vi "GetFeaturesToRegister.vi"(6 "Supported Metrics":string[](array[string]), 7 "high rate":bool, 8 "error in (no error)":errorcluster, 10 "group":string, 11 "channels":T1[](array[typedef])) -> (0 "error out":errorcluster, 2 "atleast one":bool, 3 "register trend":T5)   [LabVIEW 2017, in "McsaAnalysisHighRate.lvlib"]
uses:
  <vilib>/addons/InsightCM/Devices/Shared/Mcsa/McsaAnalysisHighRate/McsaAnalysisHighRate.lvlib
  <vilib>/addons/InsightCM/Devices/Shared/Common/DataEventCreator/controls/RegisterTrendPoints.ctl
  <vilib>/addons/InsightCM/Devices/Shared/Common/DataEventCreator/controls/Registry_Trend.ctl
  <vilib>/addons/InsightCM/Utilities/Analysis/MCSA/controls/McsaChannel.ctl
  <vilib>/addons/InsightCM/Utilities/Analysis/Shared/controls/Feature.ctl
  <vilib>/addons/InsightCM/Utilities/Analysis/Shared/controls/AmplitudeScale.ctl
  <vilib>/addons/InsightCM/MessageBus/Base/controls/KeyValuePair.ctl
  <vilib>/addons/InsightCM/Devices/Shared/Common/DataEventCreator/DataEventCreator.lvlib
  <vilib>/addons/InsightCM/Utilities/Analysis/Shared/AnalysisHelper.lvlib
  <vilib>/addons/InsightCM/Utilities/Analysis/MCSA/McsaAnalysisFunctions.lvlib
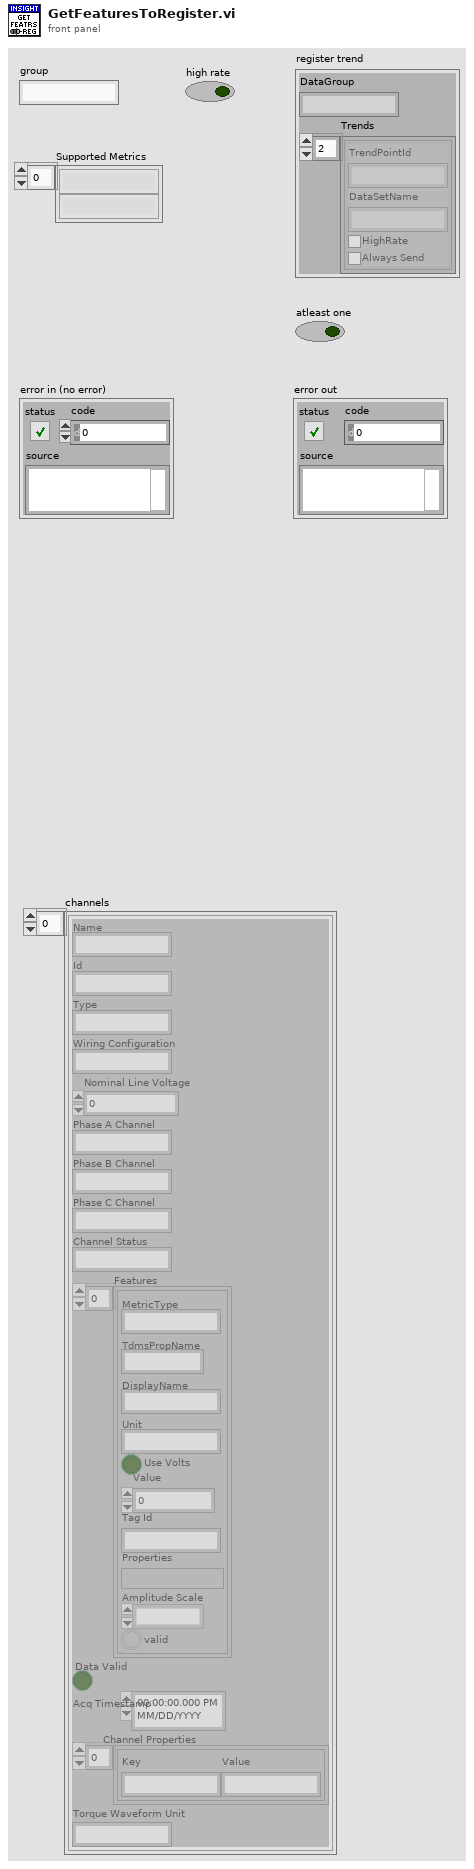
[diagram p1: front panel]
types:
  T1 = typedef "McsaAnalysisFunctions.lvlib/McsaChannel.ctl" = cluster{"Name":string, "Id":string, "Type":string, "Wiring Configuration":string, "Nominal Line Voltage":dbl, "Phase A Channel":string, "Phase B Channel":string, "Phase C Channel":string, "Channel Status":string, "Features":T2[], "Data Valid":bool, "Acq Timestamp":timestamp, "Channel Properties":T4[], "Torque Waveform Unit":string}
  T2 = typedef "AnalysisHelper.lvlib/Feature.ctl" = cluster{"MetricType":string, "TdmsPropName":string, "DisplayName":string, "Unit":string, "Use Volts":bool, "Value":dbl, "Tag Id":string, "Properties":variant, "Amplitude Scale":T3, "valid":bool}
  T3 = typedef "AnalysisHelper.lvlib/AmplitudeScale.ctl" = enum16{"rms", "peak", "pk-pk"}
  T4 = typedef "KeyValuePair.ctl" = cluster{"Key":string, "Value":string}
  T5 = typedef "DataEventCreator.lvlib/RegisterTrendPoints.ctl" = cluster{"DataGroup":string, "Trends":T6[]}
  T6 = typedef "DataEventCreator.lvlib/Registry_Trend.ctl" = cluster{"TrendPointId":string, "DataSetName":string, "HighRate":bool, "Always Send":bool}
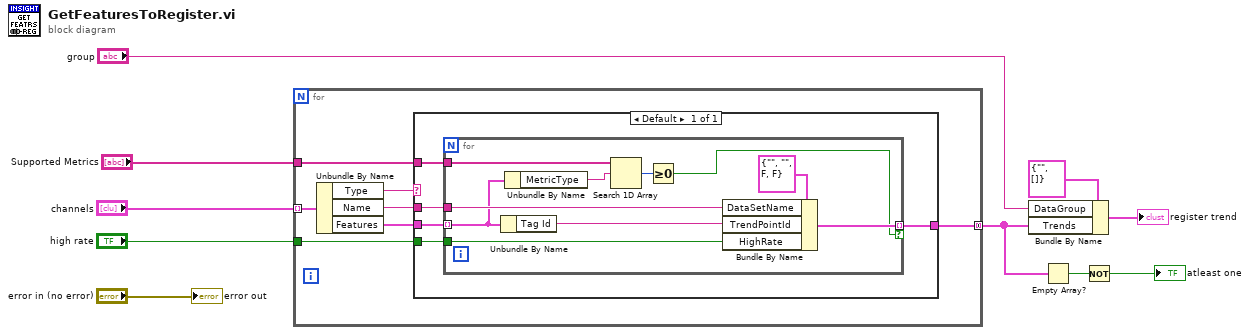
[diagram p0: block diagram]
diagram:
  n1 = for {
    tunnel: "channels" -> [w17] mode=indexing
    tunnel: [w15] -> w6 mode=concatenating
    tunnel: "high rate" -> [w12]
    tunnel: "Supported Metrics" -> [w11]
    n2 = Unbundle By Name(w17) -> ("Type"=w13:string, "Name"=w14:string, "Features"=w16:T2[])
    n3 = case shown="Default" w13 {
      tunnel: w16 -> [w22]
      tunnel: [w21] -> w15
      tunnel: w14 -> [w20]
      tunnel: w12 -> [w19]
      tunnel: w11 -> [w18]
      frame Default {
        n4 = for {
          tunnel: w22 -> [w25] mode=indexing
          tunnel: [w32] -> w21 mode=indexing if=w23
          tunnel: w20 -> [w31]
          tunnel: w19 -> [w28]
          tunnel: w18 -> [w26]
          n5 = Unbundle By Name(w25) -> ("Tag Id"=w30:string)
          n6 = Unbundle By Name(w25) -> ("MetricType"=w24:string)
          n7 = Search 1D Array(1D array=w26, element=w24) -> (index of element=w27:i32)  [unwired: 1 in]
          n8 = Greater Or Equal To 0?(x=w27) -> (x >= 0?=w23:bool)
          n9 = Bundle By Name(cluster=T6 {"TrendPointId"="", "DataSetName"="", "HighRate"=FALSE, "Always Send"=FALSE} ("Trend"), "DataSetName"=w31, "TrendPointId"=w30, "HighRate"=w28) -> (w32:T6)
        }
      }
    }
  }
  n10 = Bundle By Name(cluster=T5 {"DataGroup"="", "Trends"=[]} ("RegisterTrend"), "DataGroup"="group", "Trends"=w6) -> (→"register trend":T5)
  n11 = Empty Array?(array=w6) -> (empty?=w7:bool)
  n12 = Not(x=w7) -> (.not. x?=→"atleast one":bool)
  "error out" <- "error in (no error)"
